vi "CoffinScanPos.vi"() -> ()   [LabVIEW 2013]
uses:
  <vilib>/Utility/file.llb/Write To Spreadsheet File (DBL).vi
panel:
  out "YPosArray":dbl[](array[numeric])
  in  "Radius":dbl
  out "XPosArray":dbl[](array[numeric])
  in  "Final X":dbl
  in  "Initial X":dbl
  in  "Number of Steps":dbl
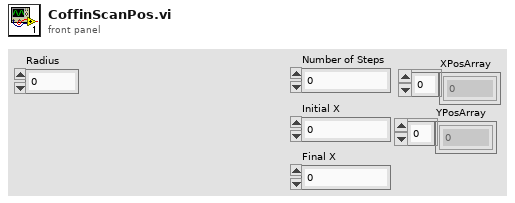
[diagram p1: front panel]
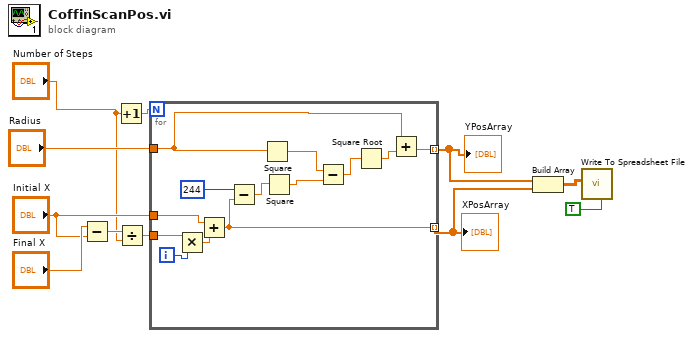
[diagram p0: block diagram]
diagram:
  n1 = Subtract(x="Final X", y="Initial X") -> (x-y=w10:dbl)
  n2 = Increment(x="Number of Steps") -> (x+1=w2:dbl)
  n3 = Divide(x=w10, y="Number of Steps") -> (x/y=w8:dbl)
  n4 = for {
    N: w2 -> [_]
    tunnel: "Initial X" -> [w24]
    tunnel: w8 -> [w22]
    tunnel: [w12] -> w6 mode=indexing
    tunnel: [w19] -> w5 mode=indexing
    tunnel: "Radius" -> [w18]
    i -> [w23]
    n5 = Multiply(x=w22, y=w23) -> (x*y=w21:dbl)
    n6 = Add(x=w24, y=w21) -> (x+y=w12:dbl)
    n7 = Subtract(x=244, y=w12) -> (x-y=w14:dbl)
    n8 = Square(x=w18) -> (x^2=w17:dbl)
    n9 = Square(x=w14) -> (x^2=w16:dbl)
    n10 = Subtract(x=w17, y=w16) -> (x-y=w15:dbl)
    n11 = Square Root(x=w15) -> (sqrt(x)=w20:dbl)
    n12 = Add(x=w18, y=w20) -> (x+y=w19:dbl)
  }
  "XPosArray" <- w6
  "YPosArray" <- w5
  n13 = Build Array(w5, w6) -> (w4:dbl[][])
  n14 = call-poly <vilib>:"Write To Spreadsheet File.vi"("transpose? (no:F)"=TRUE, "2D data"=w4) -> ()  [unwired: 6 in, 1 out]
